vi "Robot Main.vi"() -> ()   [LabVIEW 2012]
doc: "This VI imlements the framework and scheduler for your robotics program. It should not be necessary to modify the framework. You are expected to add your code to the VIs called from Robot Main, the ones located in the Team Code within the project."
uses:
  Robot Global Data.vi
panel:
  in  "Finish":bool
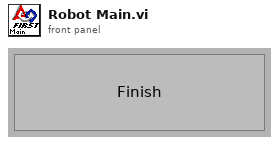
[diagram p1: front panel]
types:
  T1 = typedef "WPI_DriverStationMatch Info.ctl" = cluster{"Autonomous Elapsed Seconds":dbl, "TeleOp Elapsed Seconds":dbl, "Disabled Elapsed Seconds":dbl, "Visited Autonomous":bool, "Visited TeleOp":bool, "Visited Disabled":bool, "Autonomous Settings":cluster{"Autonomous Style":enum16{"Iterative", "Independent"}, "VI Refnum":refnum<vi>}}
  T2 = typedef "WPI_DriverStationDerivedRobotMode.ctl" = enum16{"Init", "Execute", "Stop"}
  T3 = typedef "WPI_DriverStationRobotMode2.ctl" = enum16{"Autonomous Disabled", "Autonomous Enabled", "Teleop Disabled", "Teleop Enabled", "Timeout", "Finish", "Test Disabled", "Test Enabled"}
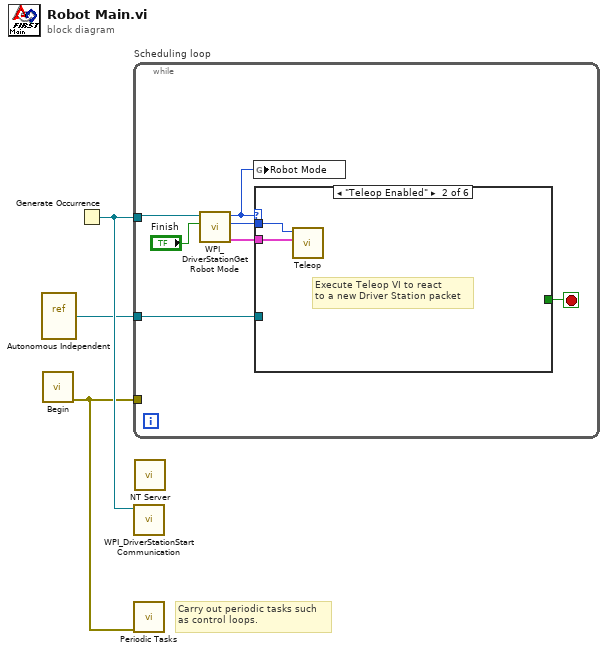
[diagram p0: block diagram]
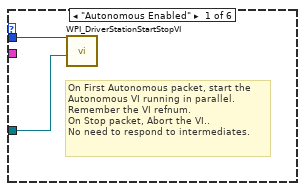
[diagram p2: hidden frame]
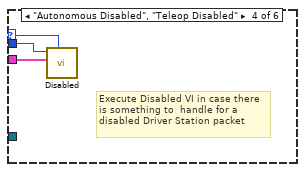
[diagram p4: hidden frame]
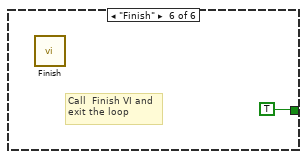
[diagram p6: hidden frame]
diagram:
  # "Carry out periodic tasks such\nas control loops."
  n1 = vi-ref "Autonomous Independent.vi"() -> (w2:refnum<vi>)
  n2 = call "Begin.vi"() -> ("error out"=w1:errorcluster)  [unwired: 1 in, 10 out]
  n3 = Generate Occurrence() -> (w3:refnum<k4>)
  n4 = while "Scheduling loop" {
    tunnel: w3 -> [w9]
    tunnel: w1 -> [_]
    tunnel: w2 -> [w5]
    stop <- w6 stop-if-true
    n5 = call <vilib>:"WPI_DriverStationGet Robot Mode.vi"("Finish"="Finish", "DS Occurrence"=w9) -> ("Match Info out"=w7:T1, "Call Context"=w10:T2, "Robot Mode"=w4:T3)  [unwired: 7 out]
    n6 = global write "Robot Global Data.vi" "Robot Mode"(w4) -> ()
    n7 = case shown="\"Teleop Enabled\"" w4 {
      selector: w4 -> [_ _ _ w15 _ _]
      tunnel: w10 -> [w12 w14 _ w17 _ _]
      tunnel: w7 -> [_ w13 _ w16 _ _]
      tunnel: [_ _ _ _ _ TRUE] -> w6
      tunnel: w5 -> [w11 _ _ _ _ _]
      frame "Autonomous Enabled" {
        # "On First Autonomous packet, start the\nAutonomous VI running in parallel.\nRemember the VI refnum.\nOn Stop packet, Abort the VI..\nNo need to respond to intermediates."
        n8 = call <vilib>:"WPI_DriverStationStartStopVI.vi"("VI in"=w11, "Call Context"=w12) -> ()  [unwired: 10 in]
      }
      frame "Teleop Enabled" {
        # "Execute Teleop VI to react\nto a new Driver Station packet"
        n9 = call "Teleop.vi"("Match Info"=w13, "Call Context"=w14) -> ()  [unwired: 1 in, 9 out]
      }
      frame "Test Disabled", "Test Enabled" {
      }
      frame "Autonomous Disabled", "Teleop Disabled" {
        # "Execute Disabled VI in case there\nis something to  handle for a\ndisabled Driver Station packet"
        n10 = call "Disabled.vi"("Robot Mode"=w15, "Match Info"=w16, "Call Context"=w17) -> ()  [unwired: 1 in, 8 out]
      }
      frame "Timeout" {
        # "Driver Station packet didn't arrive.\nPossibly useful for diagnostics"
      }
      frame "Finish" {
        # "Call  Finish VI and\nexit the loop"
        n11 = call "Finish.vi"() -> ()  [unwired: 1 in, 7 out]
      }
    }
  }
  n12 = call <vilib>:"WPI_DriverStationStart Communication.vi"("occurrence"=w3) -> ()  [unwired: 11 out]
  n13 = call "Periodic Tasks.vi"("error in"=w1) -> ()  [unwired: 1 in, 10 out]
  n14 = call <vilib>:"NT Server.vi"() -> ()  [unwired: 12 in]
